vi "Resume Panel Updates.vi"(8 "error in (no error)":errorcluster, 11 "IViewManager In":refnum<class "IViewManager.lvclass">) -> (0 "error out":errorcluster, 3 "IViewManager Out":refnum<class "IViewManager.lvclass">)   [LabVIEW 2020, in "MVA Framework.lvlib" / "IViewManager.lvlib" / "IViewManager.lvclass"]
doc: "恢复面板更新"
uses:
  IViewManager.lvclass
  IViewManager.lvclass/IViewManager.ctl
  <vilib>/ActorFramework/Message Enqueuer/Message Enqueuer.lvclass/Message Enqueuer.ctl
  <vilib>/ActorFramework/Message Enqueuer/Enqueue.vi
  IViewable/IViewable Messages/Resume Panel Updates Msg/Resume Panel Updates Msg.lvclass
  C:/Program Files/National Instruments/LabVIEW 2020/vi.lib/ActorFramework/Message/Message.lvclass
  <vilib>/ActorFramework/Message Priority Queue/Priority Enqueue.vi
  IViewable/IViewable/IViewable.lvclass
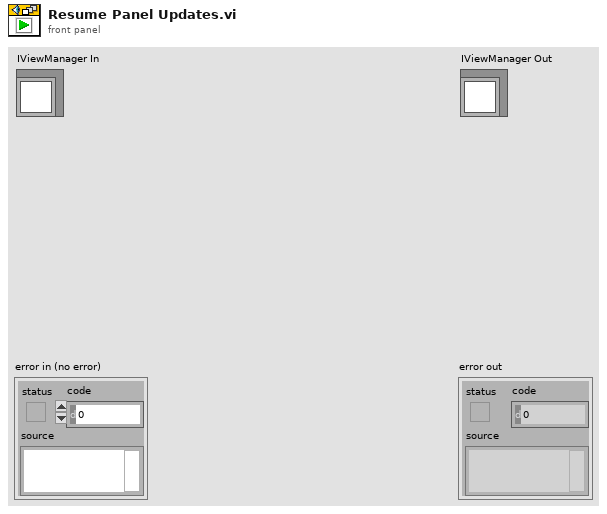
[diagram p1: front panel]
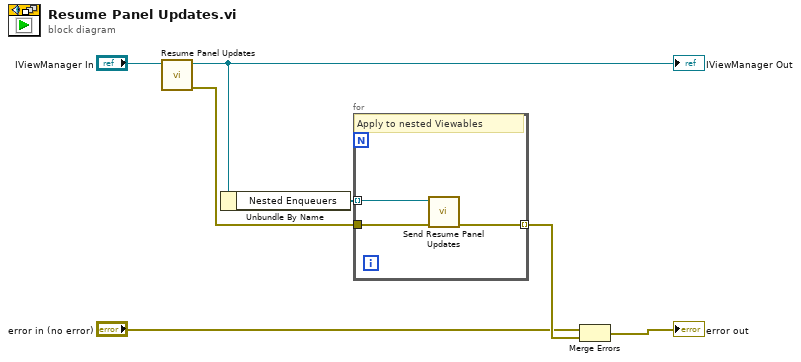
[diagram p0: block diagram]
diagram:
  n1 = call-parent "Resume Panel Updates.vi"("IViewable In"="IViewManager In") -> ("error out"=w6:errorcluster, "IViewable Out"=w1:refnum<class "IViewManager.lvclass">)  [unwired: 9 in]
  "IViewManager Out" <- w1
  n2 = Unbundle By Name(w1) -> ("Nested Enqueuers"=w7:refnum<class "Message Enqueuer.lvclass">[])
  n3 = for {
    tunnel: w7 -> [w8] mode=indexing
    tunnel: w6 -> [w10]
    tunnel: [w9] -> w5 mode=indexing
    # "Apply to nested Viewables"
    n4 = call "Send Resume Panel Updates.vi"("error in (no error)"=w10, "Message Enqueuer"=w8) -> ("error out"=w9:errorcluster)  [unwired: 8 in, 1 out]
  }
  n5 = Merge Errors("error in (no error)", w5) -> (→"error out":errorcluster)
